vi "angle_final.vi"(8 "Valeur joy":dbl, 10 "indeadzone":bool, 11 "valeur enc":dbl) -> (2 "valeur":dbl)   [LabVIEW 2015]
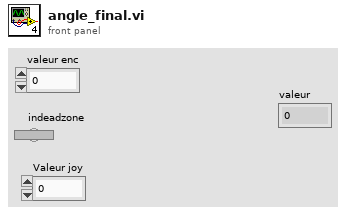
[diagram p1: front panel]
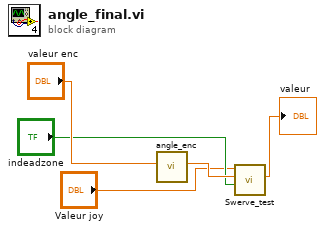
[diagram p0: block diagram]
diagram:
  n1 = call "angle_enc.vi"("encoder"="valeur enc") -> ("angle"=w5:dbl)  [unwired: 10 in]
  n2 = call "Swerve_test.vi"("indeadzone"="indeadzone", "Encoder"=w5, "Joystick"="Valeur joy") -> ("Return"=→"valeur":dbl)  [unwired: 8 in]
